vi "GET_Icon.vi"(8 "error in (no error)":errorcluster, 11 "FakedArray in":refnum<class "FakedArray.lvclass">) -> (0 "error out":errorcluster, 2 "Image":picture, 3 "FakedArray out":refnum<class "FakedArray.lvclass">)   [LabVIEW 2021, in "FakedArray.lvclass"]
uses:
  FakedArray.lvclass
  FakedArray.lvclass/FakedArray.ctl
  vi.lib/LabVIEW Icon API/lv_icon/Controls/Graphic.ctl
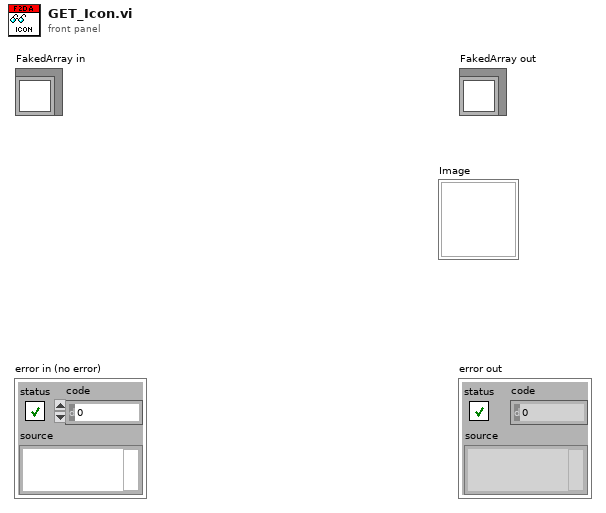
[diagram p1: front panel]
types:
  T1 = typedef "Graphic.ctl" = cluster{"Rectangle":cluster{"left":i16, "top":i16, "right":i16, "bottom":i16}, "Path":path, "Image":picture, "Filter":string, "FileName":string}
  T2 = typedef "ToMoreSpecific_Faked2DArray.ctl" = enum16{"Framework Templates", "Layer List"}
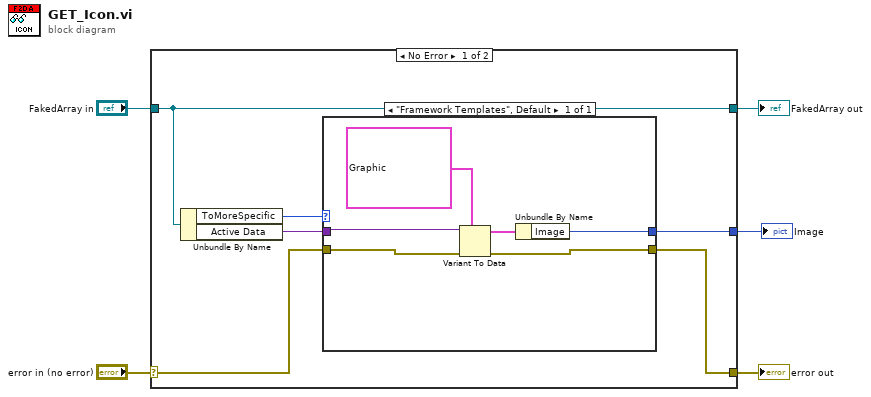
[diagram p0: block diagram]
diagram:
  n1 = case shown="No Error" "error in (no error)" {
    selector: "error in (no error)" -> [w8 w19]
    tunnel: [w7 w19] -> w4
    tunnel: [w11 w18] -> w2
    tunnel: "FakedArray in" -> [w11 w18]
    tunnel: [w6 _] -> w1
    frame No Error {
      n2 = Unbundle By Name(w11) -> ("ToMoreSpecific"=w10:T2, "Active Data"=w9:variant)
      n3 = case shown="\"Framework Templates\", Default" w10 {
        tunnel: w9 -> [w17]
        tunnel: w8 -> [w16]
        tunnel: [w15] -> w7
        tunnel: [w12] -> w6
        frame "Framework Templates", Default {
          n4 = Variant To Data(error in=w16, type=T1 {"Rectangle"={"left"=0, "top"=0, "right"=0, "bottom"=0}, "Path"=path "", "Image"=bytes[0], "Filter"="", "FileName"=""} ("Path & Icon"), Variant=w17) -> (data=w13:T1, error out=w15:errorcluster)
          n5 = Unbundle By Name(w13) -> ("Image"=w12:picture)
        }
      }
    }
    frame Error {
    }
  }
  "error out" <- w4
  "FakedArray out" <- w2
  "Image" <- w1
